vi "ITC503 -- scan ITC LTC state -- Pgg1.vi"(6 "error logfile path":path, 7 "disable interaction with itc":T1(ring)=enum."do not use oxford ITC", 8 "error in":errorcluster, 11 "state IN":T3={"LTC21 Address"="GPIB0::15::INSTR", "ITC503 Address"="GPIB0::24::INSTR", "ITC temperature"=138.96, "ITC set temperature"=55.0, "LTC temperature"=137.354, "heater"=0.0, "gas flow"=96.8, "P"=10.0, "D"=1.0, "I"=3.0, "ITC state"="X0A1C2S01H1L0\r", "nonzero temperature"=0.0, "Magn Field (T)"=0.0, "LakeShore340"="", "LS340 Adress"=0, "Sample Temperature Source"=enum."read T <- LakeShore 340", "Neocera sensor"=1, "Magnetic Field Source"=enum."none"}) -> (0 "error out":errorcluster, 1 "itc box state OUT":T2={"ITC503 Address"="GPIB0::15::INSTR", "ITC temperature"=0.0, "ITC set temperature"=300.0, "heater"=300.0, "gas flow"=1.6, "P"=0.0, "D"=10.0, "I"=0.1, "ITC state"="X0A1C2S01H1L0\r", "nonzero temperature"=0.0, "Magn Field (T)"=0.0}, 3 "state OUT":T3={"LTC21 Address"="GPIB0::15::INSTR", "ITC503 Address"="GPIB0::24::INSTR", "ITC temperature"=138.96, "ITC set temperature"=55.0, "LTC temperature"=137.354, "heater"=0.0, "gas flow"=96.8, "P"=10.0, "D"=1.0, "I"=3.0, "ITC state"="X0A1C2S01H1L0\r", "nonzero temperature"=0.0, "Magn Field (T)"=0.0, "LakeShore340"="", "LS340 Adress"=0, "Sample Temperature Source"=enum."read T <- LakeShore 340", "Neocera sensor"=1, "Magnetic Field Source"=enum."none"})   [LabVIEW 2015]
uses:
  state.ctl
  Sample_Temperature_Source_Control.ctl
  itc 503 box state.ctl
  itc 503 box - control.ctl
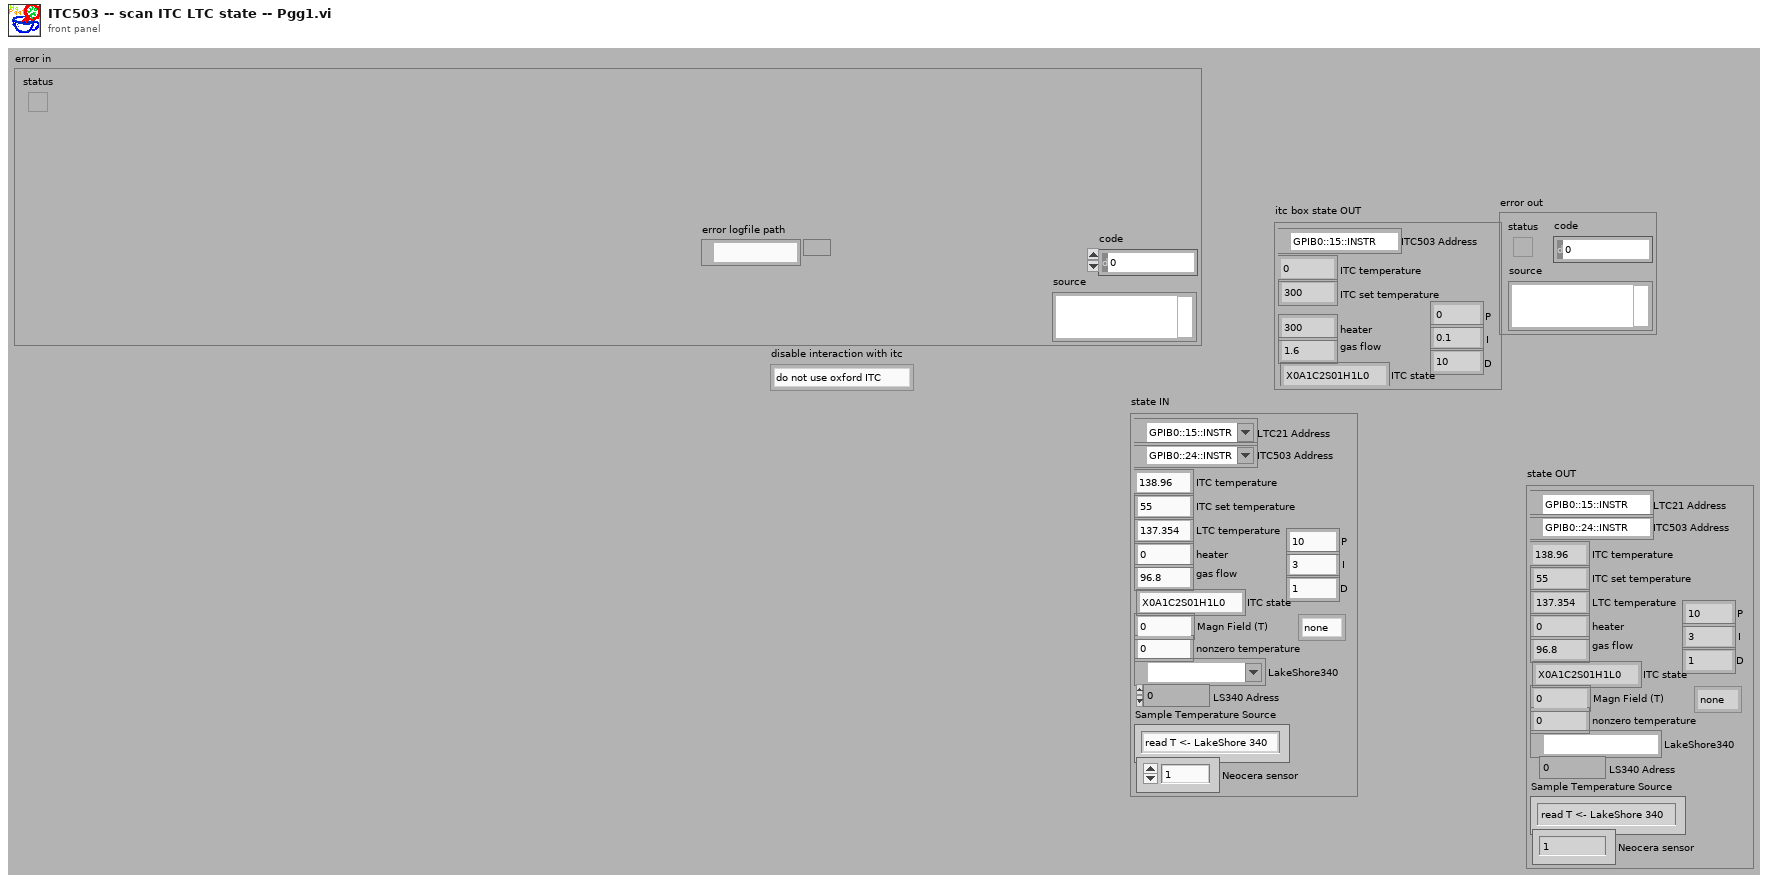
[diagram p1: front panel]
types:
  T1 = enum16{"use oxford ITC", "do not use oxford ITC"}
  T2 = typedef "itc 503 box state.ctl" = cluster{"ITC503 Address":refnum<visa-resource-name>, "ITC temperature":dbl, "ITC set temperature":dbl, "heater":dbl, "gas flow":dbl, "P":dbl, "D":dbl, "I":dbl, "ITC state":string, "nonzero temperature":dbl, "Magn Field (T)":dbl}
  T3 = typedef "state.ctl" = cluster{"LTC21 Address":refnum<visa-resource-name>, "ITC503 Address":refnum<visa-resource-name>, "ITC temperature":dbl, "ITC set temperature":dbl, "LTC temperature":dbl, "heater":dbl, "gas flow":dbl, "P":dbl, "D":dbl, "I":dbl, "ITC state":string, "nonzero temperature":dbl, "Magn Field (T)":dbl, "LakeShore340":refnum<visa-resource-name>, "LS340 Adress":i16, "Sample Temperature Source":T4, "Neocera sensor":i32, "Magnetic Field Source":enum16{"none", "20T", "Hall"}}
  T4 = typedef "Sample_Temperature_Source_Control.ctl" = enum16{"read T <- LakeShore 340", "read T <- Neocera"}
  T5 = typedef "itc 503 box - control.ctl" = enum16{"heater manual and zero", "heater auto", "upload D", "upload I", "upload P", "shut off", "init", "read sweep table", "disable", "enable", "read state", "set gas to", "stop sweep", "start sweep", "test", "set temperature to", "write sweep table", "-void", "set heater to"}
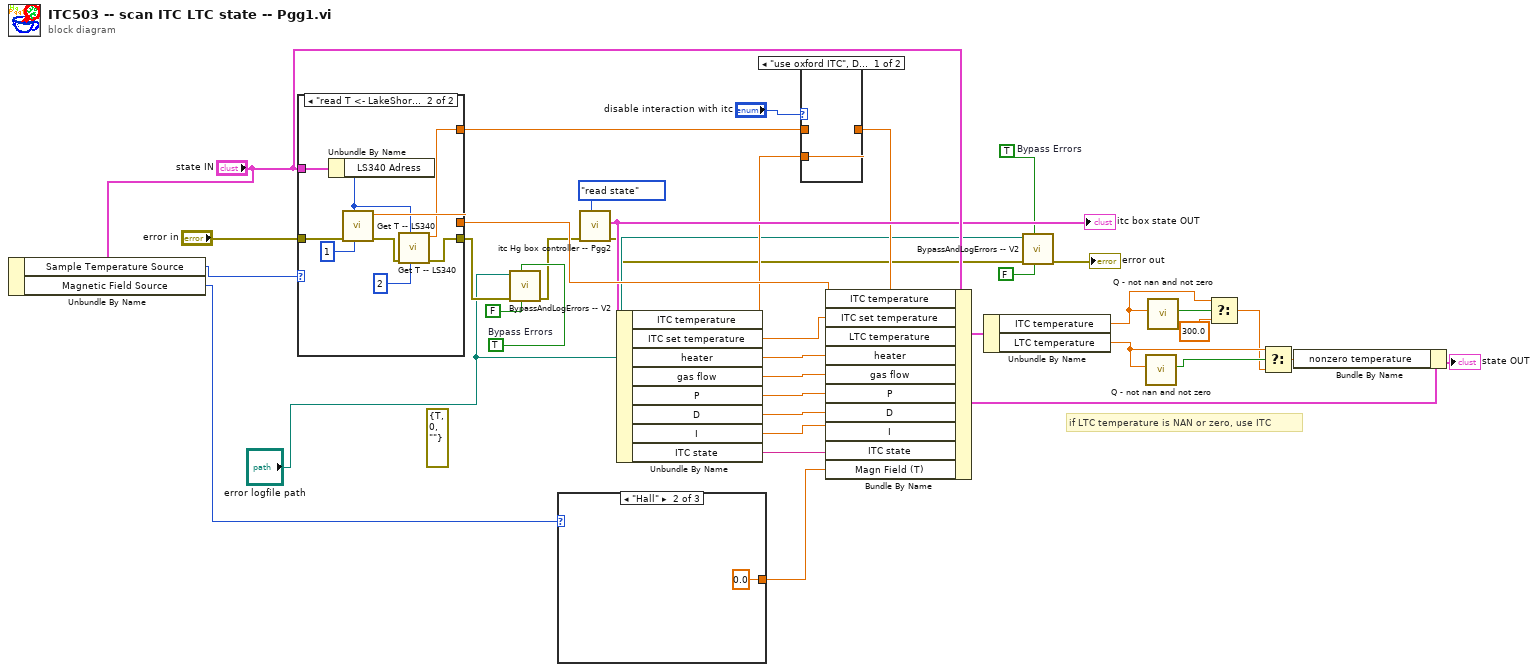
[diagram p0: block diagram]
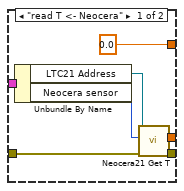
[diagram p3: hidden frame]
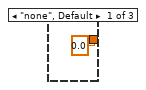
[diagram p4: hidden frame]
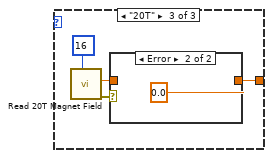
[diagram p5: hidden frame]
diagram:
  w2 = TRUE  # Bypass Errors
  w10 = TRUE  # Bypass Errors
  (unwired) errorcluster {"status"=TRUE, "code"=0, "source"=""} ("error in")
  # "if LTC temperature is NAN or zero, use ITC"
  n1 = Unbundle By Name("state IN") -> ("Sample Temperature Source"=w18:T4, "Magnetic Field Source"=w1:enum16{"none", "20T", "Hall"})
  n2 = case shown="\"read T <- LakeShore 340\"" w18 {
    tunnel: [w44 w52] -> w37
    tunnel: "state IN" -> [w43 w53]
    tunnel: "error in" -> [w42 w51]
    tunnel: [w41 w47] -> w9
    tunnel: [0.0 w45] -> w13
    frame "read T <- Neocera" {
      n3 = Unbundle By Name(w43) -> ("LTC21 Address"=w40:refnum<visa-resource-name>, "Neocera sensor"=w39:i32)
      n4 = call "Neocera21 Get T.vi"("error in (no error)"=w42, "Sensor"=w39, "VISA Resource Name"=w40) -> ("error out"=w41:errorcluster, "Temperature"=w44:dbl)  [unwired: 5 in, 2 out]
    }
    frame "read T <- LakeShore 340" {
      n5 = Unbundle By Name(w53) -> ("LS340 Adress"=w46:i16)
      n6 = call "Get T -- LS340.vi"("sensor"=1, "GPIB Adress"=w46, "error in (no error)"=w51) -> ("error out"=w48:errorcluster, "sensor Temperature"=w52:dbl)  [unwired: 6 in, 1 out]
      n7 = call "Get T -- LS340.vi"("sensor"=2, "GPIB Adress"=w46, "error in (no error)"=w48) -> ("error out"=w47:errorcluster, "sensor Temperature"=w45:dbl)  [unwired: 6 in, 1 out]
    }
  }
  n8 = call "BypassAndLogErrors -- V2.vi"("Log Error ?"=FALSE, "Bypass Errors"=w10, "error in (no error)"=w9, "Log File Path"="error logfile path") -> ("error out"=w8:errorcluster)  [unwired: 7 in]
  n9 = case shown="\"Hall\"" w1 {
    tunnel: [0.0 0.0 ("Magnetic Field (Tesla)") w56] -> w19
    frame "none", Default {
    }
    frame "Hall" {
    }
    frame "20T" {
      n10 = call "Read 20T Magnet Field.vi"("GPIB Adress"=i16 16) -> ("error out"=w58:errorcluster, "Magnetic Field (Tesla)"=w57:dbl)  [unwired: 8 in, 1 out]
      n11 = case shown="Error" w58 {
        tunnel: [w60 0.0] -> w56
        tunnel: w57 -> [w60 _]
        frame No Error {
        }
        frame Error {
        }
      }
    }
  }
  n12 = call "itc Hg box controller -- Pgg2.vi"("itc box action"=itc_503_box_-_control."read state", "error in"=w8) -> ("error out"=w4:errorcluster, "itc box state OUT"=w15:T2)  [unwired: 7 in, 1 out]
  "itc box state OUT" <- w15
  n13 = Unbundle By Name(w15) -> ("ITC temperature"=w11:dbl, "ITC set temperature"=w26:dbl, "heater"=w25:dbl, "gas flow"=w24:dbl, "P"=w23:dbl, "D"=w22:dbl, "I"=w21:dbl, "ITC state"=w20:string)
  n14 = case shown="\"use oxford ITC\", Default" "disable interaction with itc" {
    tunnel: w13 -> [_ w63]
    tunnel: [w62 w63] -> w12
    tunnel: w11 -> [w62 _]
    frame "use oxford ITC", Default {
    }
    frame "do not use oxford ITC" {
    }
  }
  n15 = Bundle By Name(cluster="state IN", "ITC temperature"=w12, "ITC set temperature"=w26, "LTC temperature"=w37, "heater"=w25, "gas flow"=w24, "P"=w23, "D"=w22, "I"=w21, "ITC state"=w20, "Magn Field (T)"=w19) -> (w35:T3)
  n16 = Unbundle By Name(w35) -> ("ITC temperature"=w30:dbl, "LTC temperature"=w32:dbl)
  n17 = call "BypassAndLogErrors -- V2.vi"("Log Error ?"=FALSE, "Bypass Errors"=w2, "error in (no error)"=w4, "Log File Path"="error logfile path") -> ("error out"=→"error out":errorcluster)  [unwired: 7 in]
  n18 = call "Q - not nan and not zero.vi"("Numeric"=w32) -> ("Boolean"=w33:bool)  [unwired: 10 in]
  n19 = call "Q - not nan and not zero.vi"("Numeric"=w30) -> ("Boolean"=w31:bool)  [unwired: 10 in]
  n20 = Select(t=w30, s=w31, f=300.0) -> (s? t:f=w28:dbl)
  n21 = Select(t=w32, s=w33, f=w28) -> (s? t:f=w27:dbl)
  n22 = Bundle By Name(cluster=w35, "nonzero temperature"=w27) -> (→"state OUT":T3)
